vi "Init Dynamic NMT.vi"() -> (1 "Inputs":T1[](array[typedef]) format="%.0x", 2 "Output":dbl[](array[numeric]))   [LabVIEW 2021]
uses:
  <vilib>/NI VeriStand/Custom Device API/Data Reference.ctl
  Global debug.vi
  <vilib>/NI VeriStand/Custom Device API/Custom Device API.lvlib
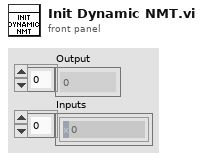
[diagram p1: front panel]
types:
  T1 = typedef "Custom Device API.lvlib/Data Reference.ctl" = i32
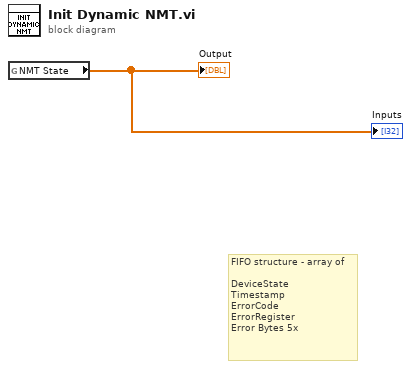
[diagram p0: block diagram]
diagram:
  # "FIFO structure - array of\n\nDeviceState\nTimestamp\nErrorCode\nErrorRegister\nError Bytes 5x"
  n1 = global read "Global debug.vi" "NMT State"() -> (→"Output" →"Inputs":dbl[])
